vi "Read Modbus.vi"(11 "Stand in":refnum<class "Stand.lvclass">) -> (2 "ModbusSp.lvclass":refnum<class "ModbusSp.lvclass">)   [LabVIEW 2019, in "Stand.lvclass"]
uses:
  Stand.lvclass
  Modbus_class/ModbusSp.lvclass
  Stand.lvclass/Stand.ctl
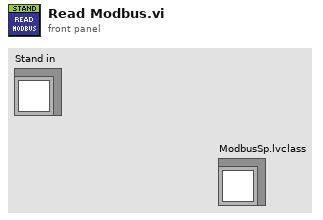
[diagram p1: front panel]
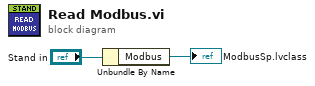
[diagram p0: block diagram]
diagram:
  n1 = Unbundle By Name("Stand in") -> ("Modbus"=→"ModbusSp.lvclass":refnum<class "ModbusSp.lvclass">)
